vi "Test Read Multiple.vi"(11 "TwinCAT ADS in":refnum<class "TwinCAT ADS.lvclass">) -> (3 "TwinCAT ADS out":refnum<class "TwinCAT ADS.lvclass">)   [LabVIEW 2018]
uses:
  TwinCAT ADS Class/TwinCAT ADS.lvclass
  Controls/Enum.ctl
  Controls/ST_Simple.ctl
  Controls/FB_Complex.ctl
  Controls/ST_Complex.ctl
  Controls/ST_Packed.ctl
  Controls/FB_Simple.ctl
  Controls/FB_Packed.ctl
  e7a7b24b-aede-49d7-b369-bb451e1de87e.vi
  TwinCAT ADS Class/VIs/Data/Read Multiple.vi
  <vilib>/addons/_JKI Toolkits/Caraya/classes/Assert/Assert Equal Value and Type_Variant.vi
  <vilib>/addons/_JKI Toolkits/Caraya/classes/Assert/Assert Equal Value_Variant.vi
  <vilib>/addons/_JKI Toolkits/Caraya/classes/Test/Test.lvclass
  <vilib>/addons/_JKI Toolkits/Caraya/classes/Assert/Assert.lvclass
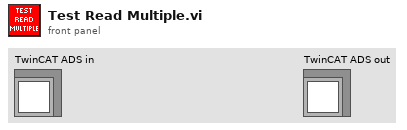
[diagram p1: front panel]
types:
  T1 = typedef "FB_Complex.ctl" = cluster{"_fMember":dbl, "_stMember":T2, "_fbSimpleMember":T6, "_fbPackedMember":T7}
  T2 = typedef "ST_Complex.ctl" = cluster{"bMember":bool, "eMember":T3, "stSimpleMember":T4, "stPackedMember":T5, "FB_Simple":T6, "arrfMember":dbl[]}
  T3 = typedef "Enum.ctl" = enum16{"Member 0", "Member 1", "Member 2"}
  T4 = typedef "ST_Simple.ctl" = cluster{"bMember":bool, "dtMember":timestamp, "nMember":i32}
  T5 = typedef "ST_Packed.ctl" = cluster{"bMember":bool, "dtMember":timestamp, "fMember":dbl}
  T6 = typedef "FB_Simple.ctl" = cluster{"_bMember":bool, "_nMember":i32, "_sMember":string}
  T7 = typedef "FB_Packed.ctl" = cluster{"bMember":bool, "nMember":i32, "sMember":string}
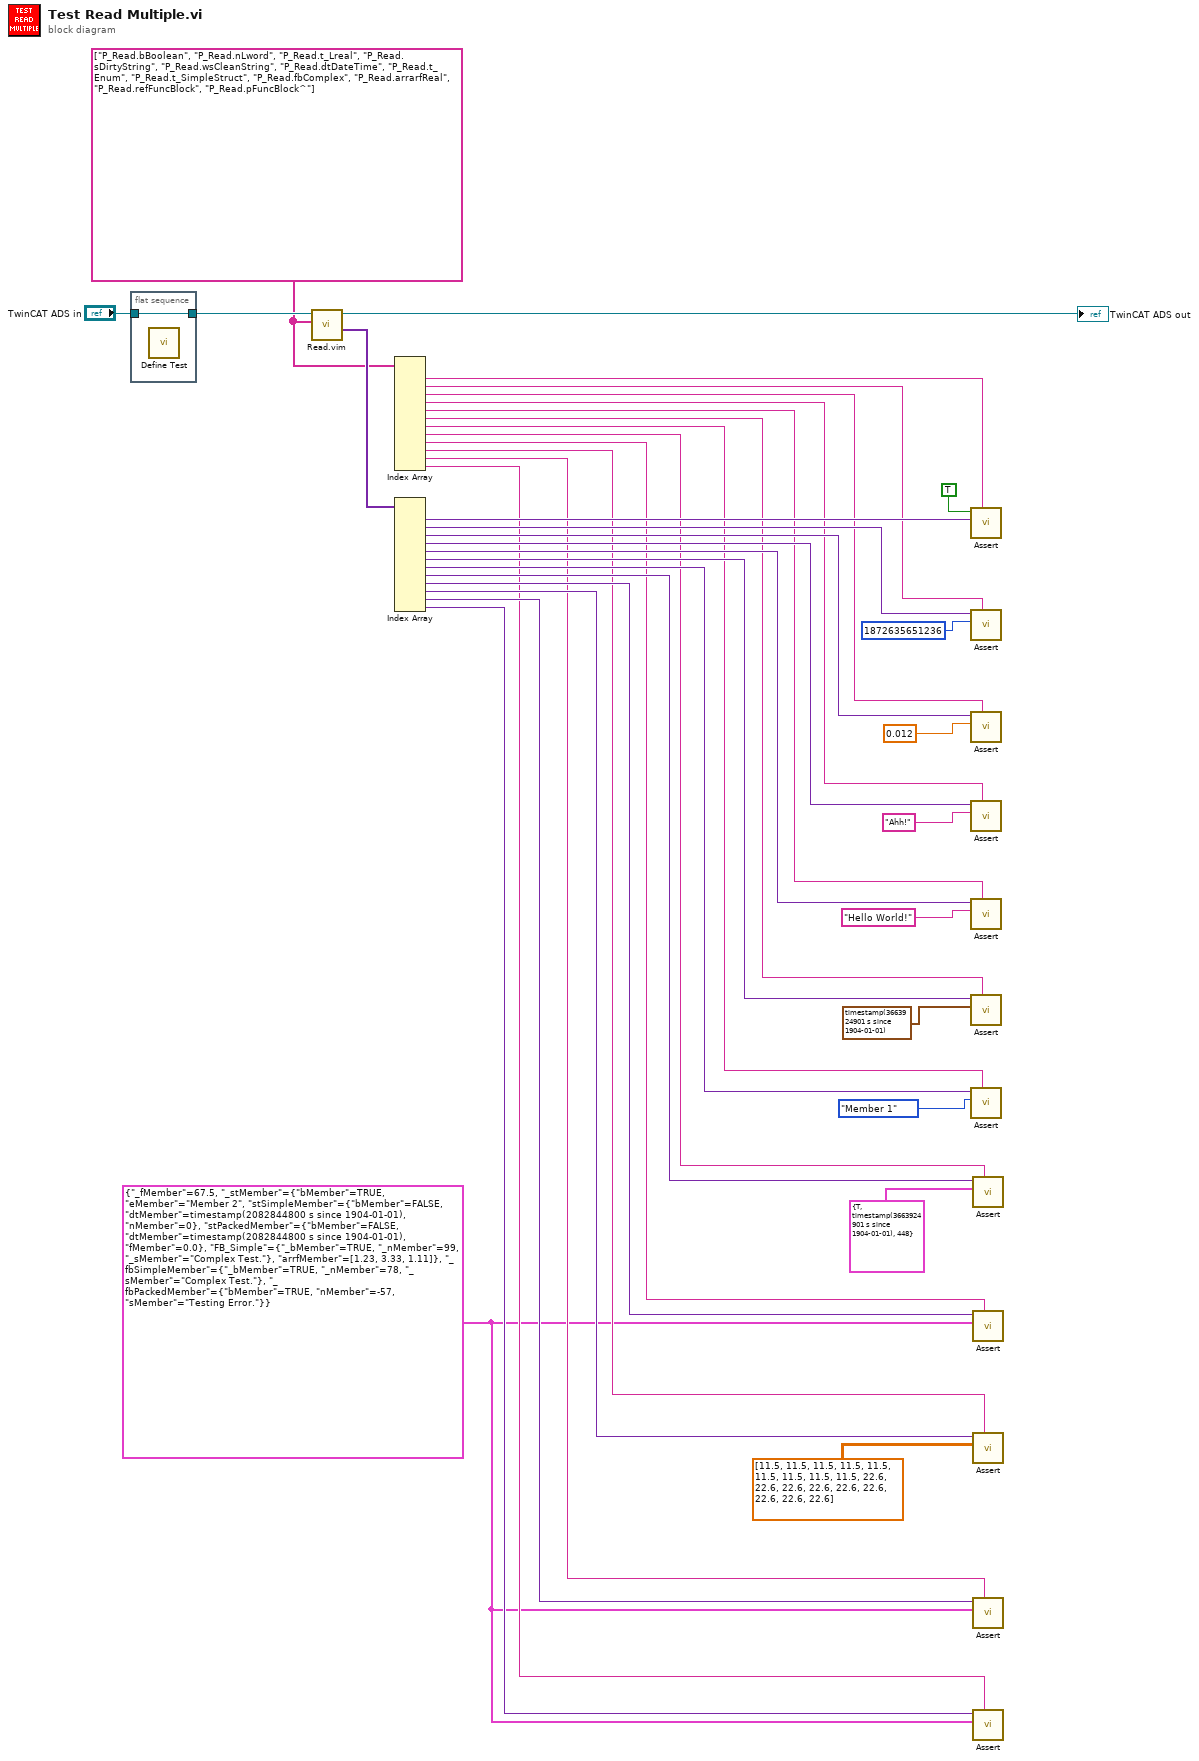
[diagram p0: block diagram]
diagram:
  w1 = T1 {"_fMember"=67.5, "_stMember"={"bMember"=TRUE, "eMember"=enum."Member 2", "stSimpleMember"={"bMember"=FALSE, "dtMember"=timestamp(2082844800 s since 1904-01-01), "nMember"=0}, "stPackedMember"={"bMember"=FALSE, "dtMember"=timestamp(2082844800 s since 1904-01-01), "fMember"=0.0}, "FB_Simple"={"_bMember"=TRUE, "_nMember"=99, "_sMember"="Complex Test."}, "arrfMember"=[1.23, 3.33, 1.11]}, "_fbSimpleMember"={"_bMember"=TRUE, "_nMember"=78, "_sMember"="Complex Test."}, "_fbPackedMember"={"bMember"=TRUE, "nMember"=-57, "sMember"="Testing Error."}} ("Value")
  w33 = string[] ["P_Read.bBoolean", "P_Read.nLword", "P_Read.t_Lreal", "P_Read.sDirtyString", "P_Read.wsCleanString", "P_Read.dtDateTime", "P_Read.t_Enum", "P_Read.t_SimpleStruct", "P_Read.fbComplex", "P_Read.arrarfReal", "P_Read.refFuncBlock", "P_Read.pFuncBlock^"]
  n1 = flat-sequence {
    tunnel: "TwinCAT ADS in" -> [w40]
    tunnel: [w40] -> w38
    frame #0 {
      n2 = call <vilib>:"Define Test.vi"() -> ()  [unwired: 10 in, 2 out]
    }
  }
  n3 = call "Read.vim"("Symbol Name"=w33, "TwinCAT ADS in"=w38) -> ("Value"=w36:variant[], "TwinCAT ADS out"=→"TwinCAT ADS out":refnum<class "TwinCAT ADS.lvclass">)  [unwired: 7 in, 1 out]
  n4 = Index Array(array=w33) -> (element #1=w32:string, element #2=w31:string, element #3=w27:string, element #4=w25:string, element #5=w21:string, element #6=w19:string, element #7=w16:string, element #8=w13:string, element #9=w10:string, element #10=w8:string, element #11=w5:string, element #12=w3:string)  [unwired: 12 in]
  n5 = Index Array(array=w36) -> (element #1=w35:variant, element #2=w30:variant, element #3=w26:variant, element #4=w24:variant, element #5=w20:variant, element #6=w18:variant, element #7=w15:variant, element #8=w12:variant, element #9=w9:variant, element #10=w6:variant, element #11=w4:variant, element #12=w2:variant)  [unwired: 12 in]
  n6 = call-poly <vilib>:"Assert.vi"("Label"=w32, "Y"=w35, "X"=TRUE) -> ()  [unwired: 7 in, 2 out]
  n7 = call-poly <vilib>:"Assert.vi"("Label"=w31, "Y"=u64 1872635651236, "X"=w30) -> ()  [unwired: 7 in, 2 out]
  n8 = call-poly <vilib>:"Assert.vi"("Label"=w27, "Y"=0.012, "X"=w26) -> ()  [unwired: 7 in, 2 out]
  n9 = call-poly <vilib>:"Assert.vi"("Label"=w25, "Y"="Ahh!", "X"=w24) -> ()  [unwired: 7 in, 2 out]
  n10 = call-poly <vilib>:"Assert.vi"("Label"=w21, "Y"="Hello World!", "X"=w20) -> ()  [unwired: 7 in, 2 out]
  n11 = call-poly <vilib>:"Assert.vi"("Label"=w19, "Y"=timestamp(3663924901 s since 1904-01-01) ("Value"), "X"=w18) -> ()  [unwired: 7 in, 2 out]
  n12 = call-poly <vilib>:"Assert.vi"("Label"=w16, "Y"=Enum."Member 1" ("Enum"), "X"=w15) -> ()  [unwired: 7 in, 2 out]
  n13 = call-poly <vilib>:"Assert.vi"("Label"=w13, "Y"=T4 {"bMember"=TRUE, "dtMember"=timestamp(3663924901 s since 1904-01-01), "nMember"=448} ("ST_Simple"), "X"=w12) -> ()  [unwired: 7 in, 2 out]
  n14 = call-poly <vilib>:"Assert.vi"("Label"=w10, "Y"=w1, "X"=w9) -> ()  [unwired: 7 in, 2 out]
  n15 = call-poly <vilib>:"Assert.vi"("Label"=w8, "Y"=dbl[][][] [[[11.5, 11.5, 11.5], [11.5, 11.5, 11.5], [11.5, 11.5, 11.5]], [[22.6, 22.6, 22.6], [22.6, 22.6, 22.6], [22.6, 22.6, 22.6]]], "X"=w6) -> ()  [unwired: 7 in, 2 out]
  n16 = call-poly <vilib>:"Assert.vi"("Label"=w5, "Y"=w1, "X"=w4) -> ()  [unwired: 7 in, 2 out]
  n17 = call-poly <vilib>:"Assert.vi"("Label"=w3, "Y"=w1, "X"=w2) -> ()  [unwired: 7 in, 2 out]
